vi "add_operation_to_SQL_pinion.vi"(4 "station_number":u16, 6 "pinion_ID":string, 8 "error_in":errorcluster, 9 "user_ID":string, 10 "save_operation_to_SQL":bool, 11 "SQL_connection_reference":T1) -> (0 "error_out":errorcluster)   [LabVIEW 2020]
uses:
  <vilib>/addons/database/Connection.llb/Conn ObjectReference.ctl
  <vilib>/addons/database/Auxilliary.llb/DB Tools Transaction.ctl
  FGV/DIAGNOSTICS_message_history_buffer/FGV_PROXY_DIAGNOSTICS_message_history_buffer.ctl
  <vilib>/addons/database/Connection.llb/Conn Transaction.vi
  <vilib>/addons/database/Connection.llb/Conn Execute.vi
  <vilib>/addons/database/Recordset.llb/Rec Destroy - Connection.vi
  <vilib>/addons/database/NI_Database_API.lvlib
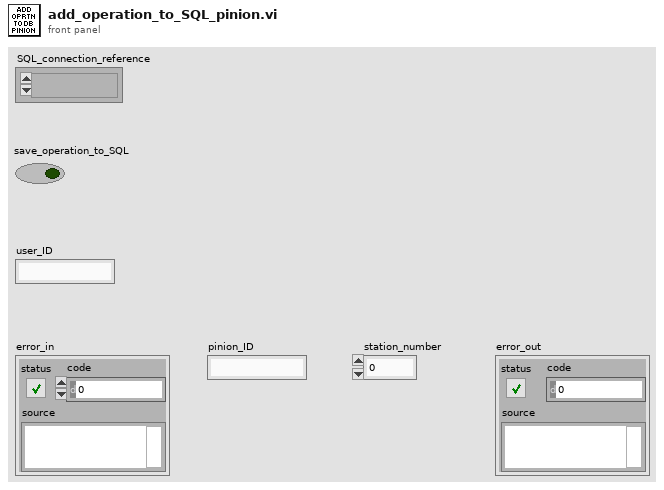
[diagram p1: front panel]
types:
  T1 = typedef "NI_Database_API.lvlib/Conn ObjectReference.ctl" = refnum<k1>
  T2 = typedef "FGV_PROXY_DIAGNOSTICS_message_history_buffer.ctl" = enum16{"initialize", "add_TCP_PLC_to_PC", "add_TCP_PC_to_PLC", "add_SQL_PC_to_DB", "add_SQL_transaction", "add_SQL_DB_to_PC", "get_station", "get_all", "clear_station", "clear_all", "save_log"}
  T3 = typedef "NI_Database_API.lvlib/DB Tools Transaction.ctl" = enum16{"begin", "commit", "rollback"}
  T4 = typedef "NI_Database_API.lvlib/Rec ObjectReference.ctl" = refnum<k1>
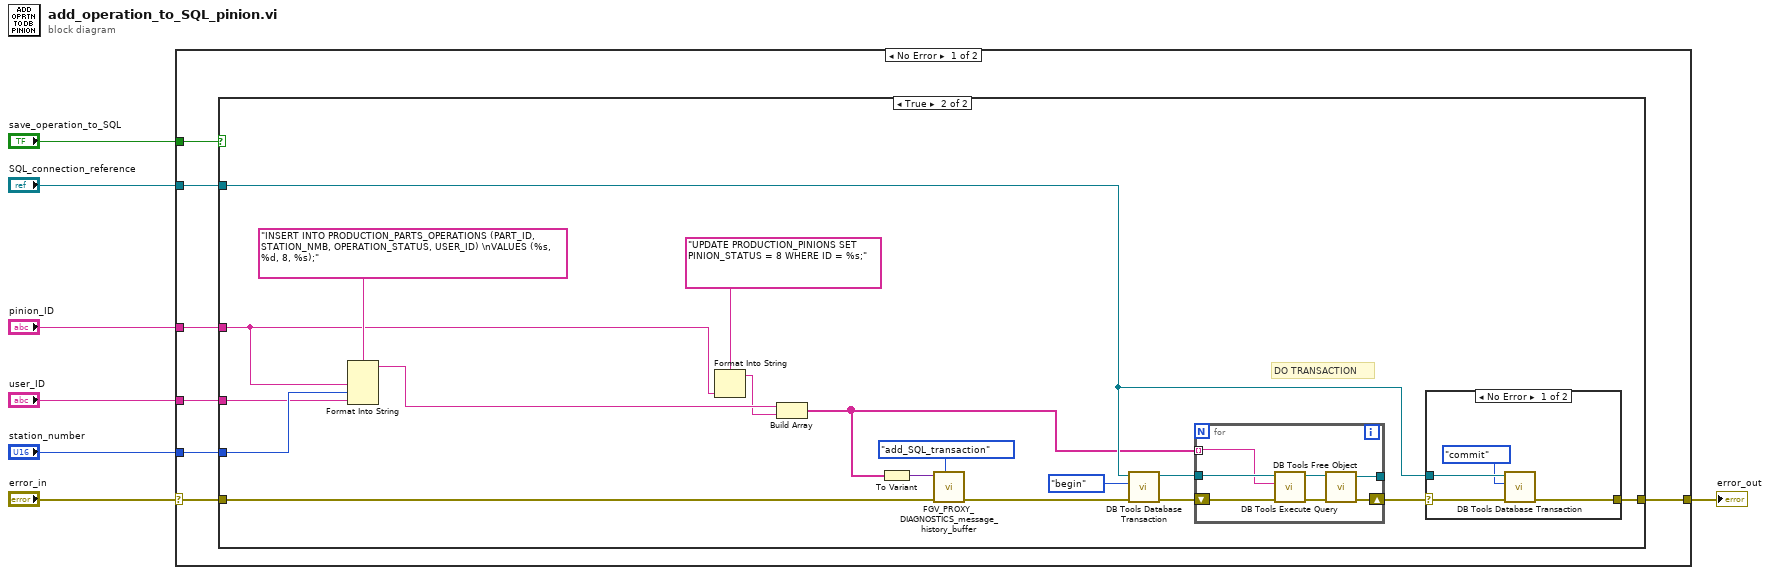
[diagram p0: block diagram]
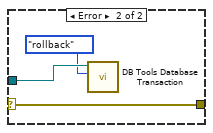
[diagram p3: hidden frame]
diagram:
  n1 = case shown="No Error" "error_in" {
    selector: "error_in" -> [w13 w48]
    tunnel: "SQL_connection_reference" -> [w14 _]
    tunnel: [w12 w48] -> w7
    tunnel: "save_operation_to_SQL" -> [w11 _]
    tunnel: "station_number" -> [w10 _]
    tunnel: "pinion_ID" -> [w9 _]
    tunnel: "user_ID" -> [w8 _]
    frame No Error {
      n2 = case shown="True" w11 {
        tunnel: w14 -> [_ w27]
        tunnel: w13 -> [w15 w19]
        tunnel: [w15 w28] -> w12
        tunnel: w10 -> [_ w25]
        tunnel: w9 -> [_ w24]
        tunnel: w8 -> [_ w16]
        frame False {
        }
        frame True {
          # "DO TRANSACTION"
          n3 = Format Into String(format string="INSERT INTO PRODUCTION_PARTS_OPERATIONS (PART_ID, STATION_NMB, OPERATION_STATUS, USER_ID) \nVALUES (%s, %d, 8, %s);", w24, w25, w16) -> (resulting string=w23:string)  [unwired: 2 in, 1 out]
          n4 = Format Into String(format string="UPDATE PRODUCTION_PINIONS SET PINION_STATUS = 8 WHERE ID = %s;", w24) -> (resulting string=w22:string)  [unwired: 2 in, 1 out]
          n5 = Build Array(w23, w22) -> (w17:string[])
          n6 = To Variant(anything=w17) -> (Variant=w21:variant)
          n7 = call "FGV_PROXY_DIAGNOSTICS_message_history_buffer.vi"("options"=FGV_PROXY_DIAGNOSTICS_message_history_buffer."add_SQL_transaction", "error_in"=w19, "input"=w21) -> ("error_out"=w18:errorcluster)  [unwired: 7 in, 1 out]
          n8 = call-poly <vilib>:"DB Tools Database Transaction.vi"("error in (no error)"=w18, "operation (begin)"=DB_Tools_Transaction."begin", "connection reference"=w27) -> ("error out"=w30:errorcluster, "connection reference out"=w31:T1)  [unwired: 3 in]
          n9 = for {
            tunnel: w31 -> [w37]
            tunnel: [w35] -> _
            shift-right: [w36] -> w32
            shift-left: w30 -> [w38]
            tunnel: w17 -> [w34] mode=indexing
            n10 = call-poly <vilib>:"DB Tools Execute Query.vi"("error in (no error)"=w38, "SQL query"=w34, "connection reference"=w37) -> ("error out"=w39:errorcluster, "recordset reference"=w40:T4)  [unwired: 5 in]
            n11 = call-poly <vilib>:"DB Tools Free Object.vi"("error in (no error)"=w39, "recordset reference"=w40) -> ("error out"=w36:errorcluster, "connection reference"=w35:T1)  [unwired: 8 in]
          }
          n12 = case shown="No Error" w32 {
            selector: w32 -> [w42 w45]
            tunnel: w27 -> [w44 w47]
            tunnel: [w41 w45] -> w28
            frame No Error {
              n13 = call-poly <vilib>:"DB Tools Database Transaction.vi"("error in (no error)"=w42, "operation (begin)"=DB_Tools_Transaction."commit", "connection reference"=w44) -> ("error out"=w41:errorcluster)  [unwired: 3 in, 1 out]
            }
            frame Error {
              n14 = call-poly <vilib>:"DB Tools Database Transaction.vi"("operation (begin)"=DB_Tools_Transaction."rollback", "connection reference"=w47) -> ()  [unwired: 4 in, 2 out]
            }
          }
        }
      }
    }
    frame Error {
    }
  }
  "error_out" <- w7
